vi "3.2.vi"() -> ()   [LabVIEW 2017]
panel:
  out "平均 2":dbl
  out "最小 2":dbl
  out "最大 2":dbl
  out "平均值":cluster{dbl, dbl}(graph)
  in  "长按停止":bool
  # "任务二"
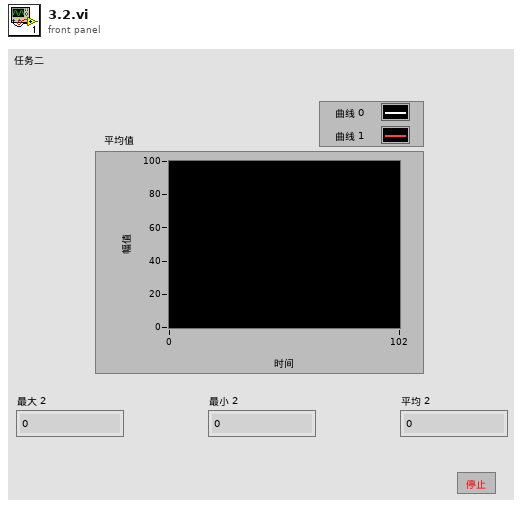
[diagram p1: front panel]
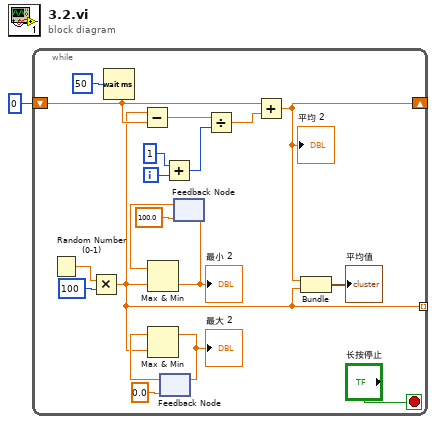
[diagram p0: block diagram]
diagram:
  n1 = while {
    shift-right: [w10] -> _
    shift-left: 0 -> [w13]
    tunnel: [w4] -> _ mode=indexing
    i -> [w14]
    stop <- "长按停止" stop-if-true
    n2 = Random Number (0-1)() -> (number: 0 to 1=w19:dbl)
    n3 = Multiply(x=w19, y=100) -> (x*y=w4:dbl)
    n4 = Wait (ms)(milliseconds to wait=u32 50 ("毫秒计时值")) -> ()  [unwired: 1 out]
    n5 = Subtract(x=w4, y=w13) -> (x-y=w16:dbl)
    n6 = feedback #1(0.0) -> (w5:dbl)
    n7 = Max & Min(x=w5, y=w4) -> (max(x,y)=w7:dbl)  [unwired: 1 out]
    "最大 2" <- w7
    n8 = feedback-in #1(w7) -> ()
    n9 = Add(x=1, y=w14) -> (x+y=w17:i32)
    n10 = feedback #2(100.0) -> (w9:dbl)
    n11 = Max & Min(x=w9, y=w4) -> (min(x,y)=w6:dbl)  [unwired: 1 out]
    "最小 2" <- w6
    n12 = feedback-in #2(w6) -> ()
    n13 = Divide(x=w16, y=w17) -> (x/y=w18:dbl)
    n14 = Add(x=w13, y=w18) -> (x+y=w10:dbl)
    "平均 2" <- w10
    n15 = Bundle(w10, w4) -> (→"平均值":cluster{dbl, dbl})  [unwired: 1 in]
  }
